vi "Configuration-GetAll.vi"(7 "error in (no error)":errorcluster caption="错误输入（无错误）") -> (0 "error IO":errorcluster)   [LabVIEW 2014]
uses:
  Configuration-Global.vi
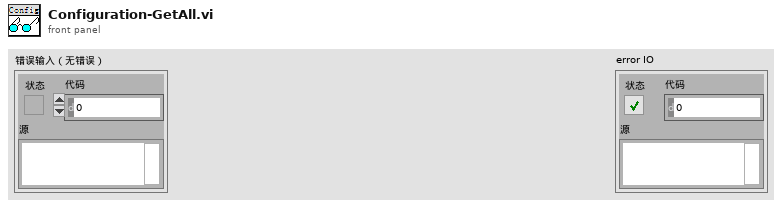
[diagram p1: front panel]
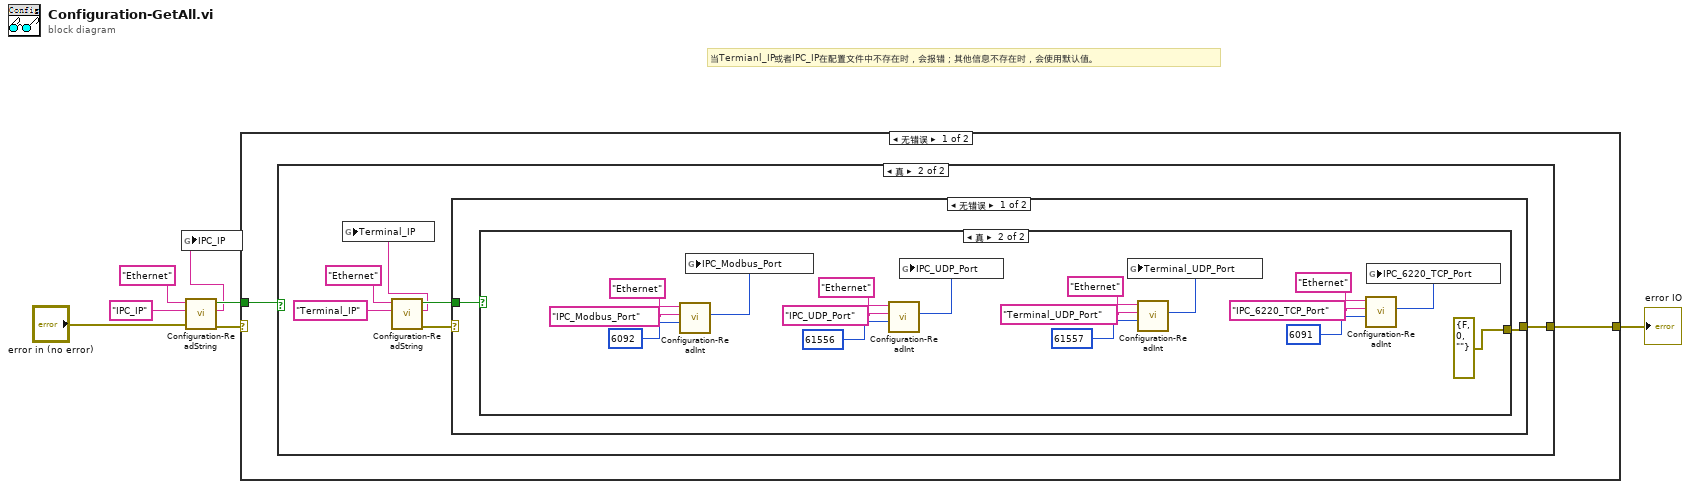
[diagram p0: block diagram]
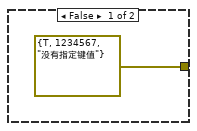
[diagram p2: hidden frame]
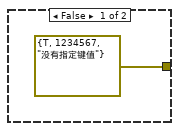
[diagram p3: hidden frame]
diagram:
  # "当Termianl_IP或者IPC_IP在配置文件中不存在时，会报错；其他信息不存在时，会使用默认值。"
  n1 = call "Configuration-ReadString.vi"("error in (no error)"="error in (no error)", "key"="IPC_IP", "section"="Ethernet") -> ("error out"=w5:errorcluster, "value"=w3:string, "found?"=w4:bool)  [unwired: 5 in]
  n2 = global write "Configuration-Global.vi" "IPC_IP"(w3) -> ()
  n3 = case shown="无错误" w5 {
    selector: w5 -> [_ w38]
    tunnel: w4 -> [w9 _]
    tunnel: [w8 w38] -> w2
    frame No Error {
      n4 = case shown="真" w9 {
        tunnel: [errorcluster {"status"=TRUE, "code"=1234567, "source"="没有指定键值"} ("错误常量") w11] -> w8
        frame False {
        }
        frame True {
          n5 = call "Configuration-ReadString.vi"("key"="Terminal_IP", "section"="Ethernet") -> ("error out"=w14:errorcluster, "value"=w12:string, "found?"=w13:bool)  [unwired: 6 in]
          n6 = global write "Configuration-Global.vi" "Terminal_IP"(w12) -> ()
          n7 = case shown="无错误" w14 {
            selector: w14 -> [_ w37]
            tunnel: w13 -> [w18 _]
            tunnel: [w17 w37] -> w11
            frame No Error {
              n8 = case shown="真" w18 {
                tunnel: [errorcluster {"status"=TRUE, "code"=1234567, "source"="没有指定键值"} ("错误常量") errorcluster {"status"=FALSE, "code"=0, "source"=""} ("错误常量")] -> w17
                frame False {
                }
                frame True {
                  n9 = call "Configuration-ReadInt.vi"("default value"=6092, "key"="IPC_Modbus_Port", "section"="Ethernet") -> ("value"=w24:i32)  [unwired: 5 in, 2 out]
                  n10 = global write "Configuration-Global.vi" "IPC_Modbus_Port"(w24) -> ()
                  n11 = call "Configuration-ReadInt.vi"("default value"=61556, "key"="IPC_UDP_Port", "section"="Ethernet") -> ("value"=w23:i32)  [unwired: 5 in, 2 out]
                  n12 = global write "Configuration-Global.vi" "IPC_UDP_Port"(w23) -> ()
                  n13 = call "Configuration-ReadInt.vi"("default value"=61557, "key"="Terminal_UDP_Port", "section"="Ethernet") -> ("value"=w22:i32)  [unwired: 5 in, 2 out]
                  n14 = global write "Configuration-Global.vi" "Terminal_UDP_Port"(w22) -> ()
                  n15 = call "Configuration-ReadInt.vi"("default value"=6091, "key"="IPC_6220_TCP_Port", "section"="Ethernet") -> ("value"=w21:i32)  [unwired: 5 in, 2 out]
                  n16 = global write "Configuration-Global.vi" "IPC_6220_TCP_Port"(w21) -> ()
                }
              }
            }
            frame Error {
            }
          }
        }
      }
    }
    frame Error {
    }
  }
  "error IO" <- w2
